vi "WPI_UtilitiesTimebaseConstants.vi"() -> (4 "40 MHz FPGA clock":dbl=2.5e-08, 6 "1 MHz PWM clock":dbl=1e-06, 8 "500 kHz AI max clock":dbl=2e-06)   [LabVIEW 2025]
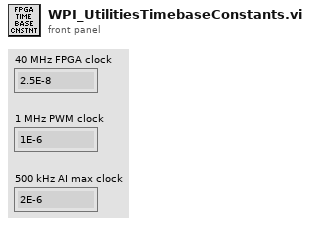
[diagram p1: front panel]
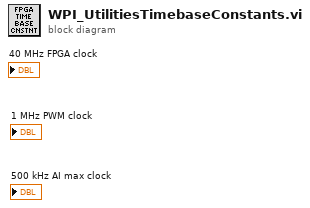
[diagram p0: block diagram]
diagram:
